vi "serialTest.vi"() -> ()   [LabVIEW 2022 SP3]
panel:
  out "Reply":string
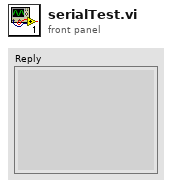
[diagram p1: front panel]
types:
  T1 = typedef "PythonCtrl.ctl" = cluster{"session":refnum<k35>, "PyPath":path, "Processor":T2, "Port":string, "version":string}
  T2 = typedef "Processors.ctl" = enum16{"SPIKE", "Pi", "Pi_ssh", "OpenMV", "Dunio"}
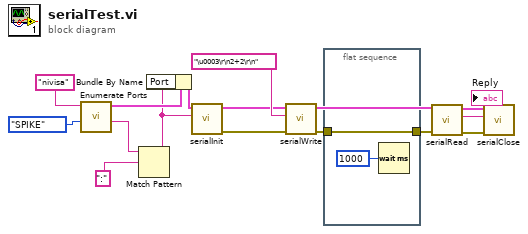
[diagram p0: block diagram]
diagram:
  n1 = call "Enumerate Ports.vi"("Processor"=enum16{"SPIKE", "Pi", "Pi_ssh"}."SPIKE", "Python version"="nivisa") -> ("guess"=w5:string, "Python"=w3:T1)  [unwired: 5 in, 3 out]
  n2 = Match Pattern(string=w5, regular expression=":") -> (before substring=w1:string)  [unwired: 1 in, 3 out]
  n3 = Bundle By Name(cluster=w3, "Port"=w1) -> (w2:T1)
  n4 = call "serialInit.vi"("Port"=w1, "Python"=w2) -> ("error out"=w14:errorcluster)  [unwired: 7 in, 2 out]
  n5 = call "serialWrite.vi"("error in (no error)"=w14, "text"="\u0003\r\n2+2\r\n", "Python"=w2) -> ("error out"=w8:errorcluster)  [unwired: 6 in, 2 out]
  n6 = flat-sequence {
    tunnel: [w15] -> w9
    tunnel: w8 -> [w15]
    frame #0 {
      n7 = Wait (ms)(milliseconds to wait=u32 1000) -> ()  [unwired: 1 out]
    }
  }
  n8 = call "serialRead.vi"("error in (no error)"=w9, "Python"=w2) -> ("error out"=w13:errorcluster, "Reply"=→"Reply":string, "Python out"=w12:T1)  [unwired: 7 in]
  n9 = call "serialClose.vi"("error in (no error)"=w13, "Python in"=w12) -> ()  [unwired: 8 in, 2 out]
